vi "fitParameterCoarseEstimate.vi"(1 "erroIn":errorcluster, 2 "Y":dbl[](array[numeric])=[2.0, 2.0, 3.0, 4.0, 5.0, 4.0, 3.0, 2.0, 2.0, 2.0], 3 "X":dbl[](array[numeric]), 4 "previousPars":dbl[](array[numeric])=[0.0, 0.0, 0.0, 0.0]) -> (0 "pars":dbl[](array[numeric]))   [LabVIEW 2021]
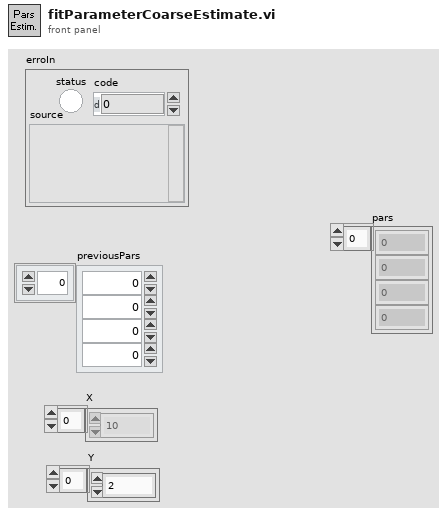
[diagram p1: front panel]
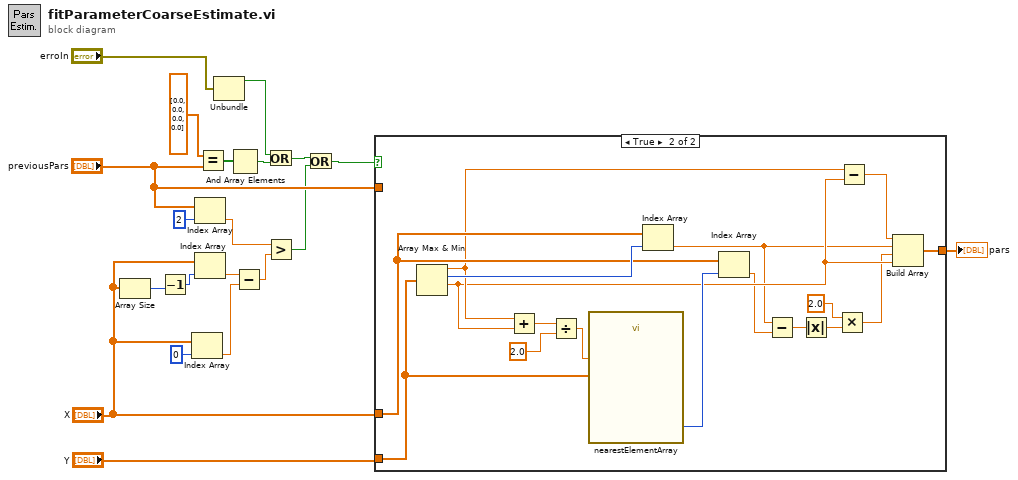
[diagram p0: block diagram]
diagram:
  n1 = Array Size(array="X") -> (size(s)=w10:i32)
  n2 = Decrement(x=w10) -> (x-1=w8:i32)
  n3 = Index Array(array="X", index=0) -> (element=w6:dbl)
  n4 = Index Array(array="previousPars", index=2) -> (element=w5:dbl)
  n5 = Index Array(array="X", index=w8) -> (element=w7:dbl)
  n6 = Equal?(x=dbl[] [0.0, 0.0, 0.0, 0.0], y="previousPars") -> (x = y?=w18:bool[])
  n7 = Unbundle("erroIn") -> ("status"=w15:bool)  [unwired: 2 out]
  n8 = And Array Elements(Boolean array=w18) -> (logical AND=w14:bool)
  n9 = Subtract(x=w7, y=w6) -> (x-y=w4:dbl)
  n10 = Or(x=w15, y=w14) -> (x .or. y?=w3:bool)
  n11 = Greater?(x=w5, y=w4) -> (0:w2:bool)
  n12 = Or(x=w3, y=w2) -> (x .or. y?=w1:bool)
  n13 = case shown="True" w1 {
    tunnel: "Y" -> [_ w38]
    tunnel: "X" -> [_ w33]
    tunnel: [w21 w22] -> w17
    tunnel: "previousPars" -> [w21 _]
    frame False {
    }
    frame True {
      n14 = Array Max & Min(array=w38) -> (max value=w31:dbl, max index (indices)=w34:i32, min value=w29:dbl)  [unwired: 1 out]
      n15 = Add(x=w31, y=w29) -> (x+y=w37:dbl)
      n16 = Divide(x=w37, y=2.0) -> (x/y=w35:dbl)
      n17 = call "nearestElementArray.vi"("value"=w35, "1D Array"=w38) -> ("index"=w32:i32)  [unwired: 8 in, 1 out]
      n18 = Index Array(array=w33, index=w34) -> (element=w28:dbl)
      n19 = Index Array(array=w33, index=w32) -> (element=w27:dbl)
      n20 = Subtract(x=w28, y=w27) -> (x-y=w26:dbl)
      n21 = Absolute Value(x=w26) -> (abs(x)=w25:dbl)
      n22 = Multiply(x=2.0, y=w25) -> (x*y=w24:dbl)
      n23 = Subtract(x=w31, y=w29) -> (x-y=w30:dbl)
      n24 = Build Array(w30, w28, w24, w29) -> (w22:dbl[])
    }
  }
  "pars" <- w17
